vi "update_raps.vi"(8 "error in (no error)":errorcluster, 10 "settings cluster":T1={"number of pixels"=0, "iterations per pixel"=0, "iterations per subpixel"=0, "maximum bit-depth"=0, "AOD center freq. (Hz)"=0.0, "AOD bandwidth freq. (Hz)"=0.0, "AOD amplitude"=0, "pixel dwell time"=0.0, "AOD equilibration time"=65535.0, "ra trajectory pixels (data/pixels transfered)"=1, "pattern type"=-1, "ellipsoid parameter cluster"={"a"=0.0, "b"=0.0, "c"=0.0, "d"=0.0, "e"=0.0, "k"=0, "width"=0.0}, "pixel values cluster"={"channel 0"=0, "channel 1"=0, "channel 2"=0, "channel 3"=0}, "offset (Hz)"=[], "RAPS array"=[], "DDS board initialization parameters"={"Bypass PLL"=FALSE, "PLL Range"=FALSE, "Update Clock"=FALSE, "Triangle "=FALSE, "SDO Active"=FALSE, "LSB First"=FALSE, "OSK Int"=FALSE, "Output Shaped Keying Enable"=FALSE, "Bypass Sinc"=FALSE, "Digital Part"=FALSE, "OutPut DAC"=FALSE, "Control DAC"=FALSE, "Comparator"=FALSE, "Modus"=0, "Multiplier Value"=0}, "gates"=[]} {"ellipsoid parameter cluster"."a" format="%.16g"; "ellipsoid parameter cluster"."b" format="%.16g"; "ellipsoid parameter cluster"."c" format="%.16g"; "ellipsoid parameter cluster"."d" format="%.16g"; "DDS board initialization parameters"."Modus" scale=0.0..4.0}, 11 "FPGA VI Reference In":refnum<k20>) -> (0 "error out":errorcluster)   [LabVIEW 2010]
uses:
  <vilib>/rvi/interface/nirviReadWriteControl/nirviReadWriteControl.xnode
  <vilib>/rvi/interface/nirviMethod/nirviMethod.xnode
  common_typedefs/channels_cluster.ctl
  fpgaVIsAndControls/DDS_board_init_cluster.ctl
  FPGAWrapperMH120124RAPS_PXI7813R/settings_cluster_raps.ctl
  fpgaVIsAndControls/ellipsoid_parameters_cluster.ctl
  common_typedefs/gate_parameters_cluster.ctl
  fpgaVIsAndControls/gate_cluster.ctl
panel:
  # "FSK"
  # "Ramped"
  # "FSK"
  # "Chirp Modus"
  # "Unramped"
  # "BPSK"
  # "Single Tone"
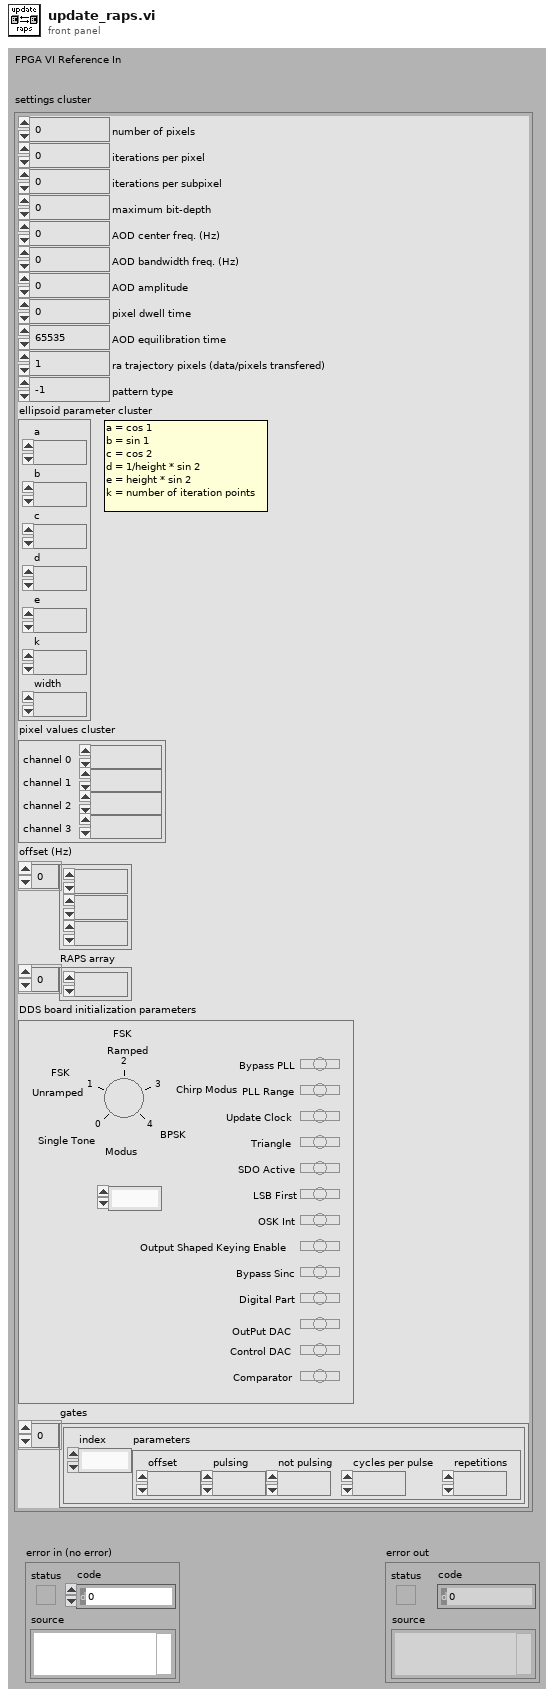
[diagram p1: front panel]
types:
  T1 = typedef "settings_cluster_raps.ctl" = cluster{"number of pixels":i32, "iterations per pixel":i32, "iterations per subpixel":i32, "maximum bit-depth":i8, "AOD center freq. (Hz)":dbl, "AOD bandwidth freq. (Hz)":dbl, "AOD amplitude":u16, "pixel dwell time":dbl, "AOD equilibration time":dbl, "ra trajectory pixels (data/pixels transfered)":u32, "pattern type":i8, "ellipsoid parameter cluster":T2, "pixel values cluster":T3, "offset (Hz)":dbl[], "RAPS array":u64[], "DDS board initialization parameters":T4, "gates":T5[]}
  T2 = typedef "ellipsoid_parameters_cluster.ctl" = cluster{"a":fxp<+/-,16,1>, "b":fxp<+/-,16,1>, "c":fxp<+/-,16,1>, "d":fxp<+/-,16,1>, "e":fxp<+/-,24,16>, "k":u16, "width":fxp<+,16,16>}
  T3 = typedef "channels_cluster.ctl" = cluster{"channel 0":u32, "channel 1":u32, "channel 2":u32, "channel 3":u32}
  T4 = typedef "DDS_board_init_cluster.ctl" = cluster{"Bypass PLL":bool, "PLL Range":bool, "Update Clock":bool, "Triangle ":bool, "SDO Active":bool, "LSB First":bool, "OSK Int":bool, "Output Shaped Keying Enable":bool, "Bypass Sinc":bool, "Digital Part":bool, "OutPut DAC":bool, "Control DAC":bool, "Comparator":bool, "Modus":u8, "Multiplier Value":u8}
  T5 = typedef "gate_cluster.ctl" = cluster{"index":i32, "parameters":T6}
  T6 = typedef "gate_parameters_cluster.ctl" = cluster{"offset":i64, "pulsing":i64, "not pulsing":i64, "cycles per pulse":i64, "repetitions":i64}
  T7 = cluster{"AOD Bandwidth_x (Hz)":fxp<+,36,32>, "AOD Bandwidth_y (Hz)":fxp<+,36,32>, "AOD half bandwidth_x":fxp<+,36,32>, "AOD half bandwidth_y":fxp<+,36,32>, "AOD_Scale_Factor (1/Zoom)":fxp<+,36,2>, "sin Phi":fxp<+/-,36,2>, "cos Phi":fxp<+/-,36,2>, "Bandwidth for LUTs (256pts)":fxp<+,36,0>, "AOD_Amplitude in":u16, "AOD center frequ. (Hz)_x":fxp<+,36,32>, "AOD center frequ. (Hz)_y":fxp<+,36,32>, "x offset (Hz)":fxp<+/-,36,32>, "y offset (Hz)":fxp<+/-,36,32>, "DA multiplier constant":fxp<+,64,4>}
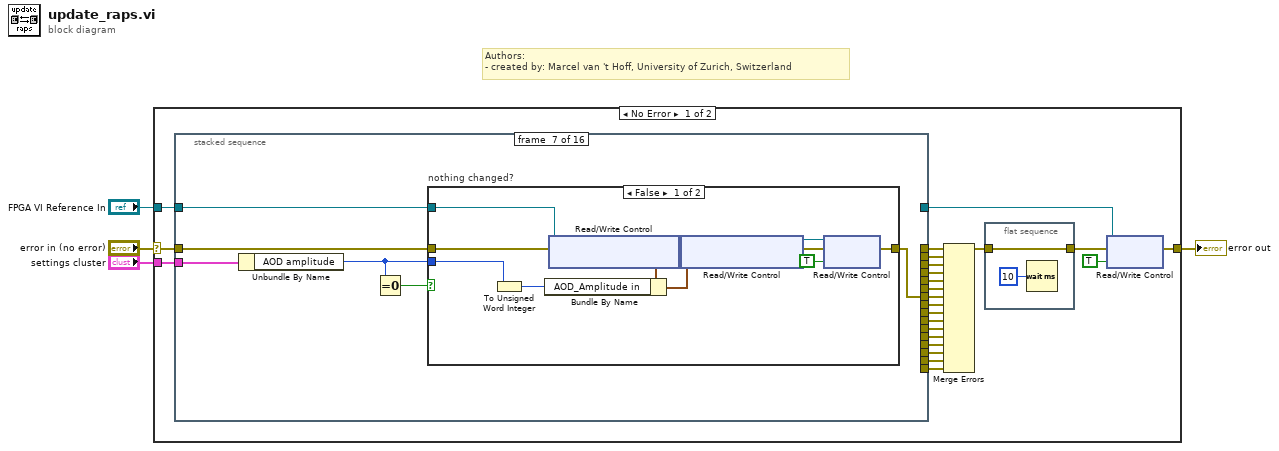
[diagram p0: block diagram]
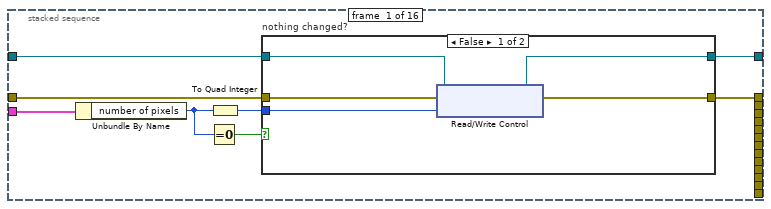
[diagram p2: hidden frame]
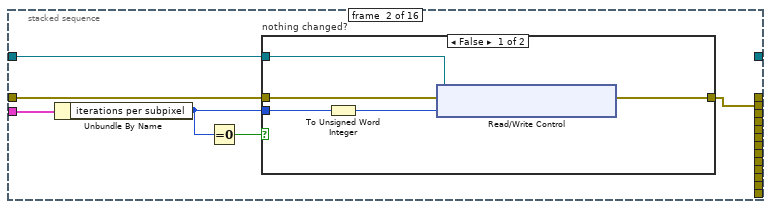
[diagram p4: hidden frame]
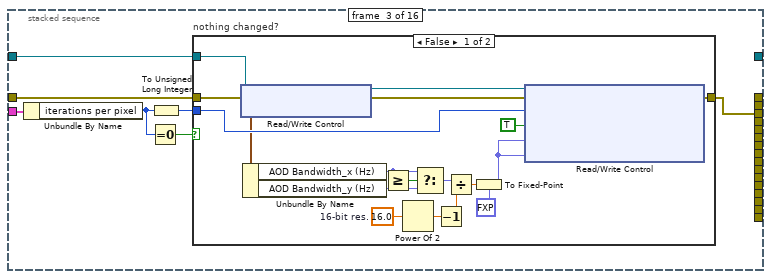
[diagram p6: hidden frame]
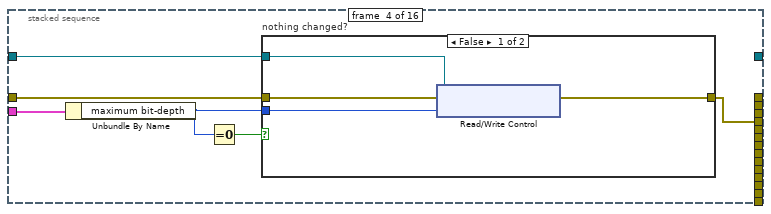
[diagram p8: hidden frame]
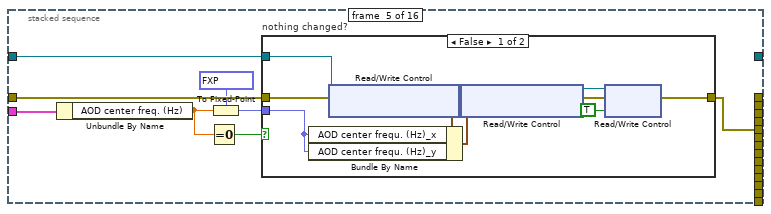
[diagram p10: hidden frame]
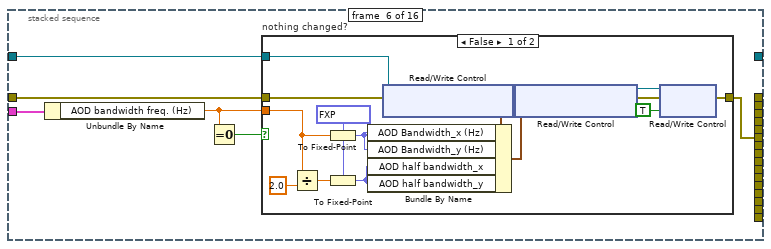
[diagram p12: hidden frame]
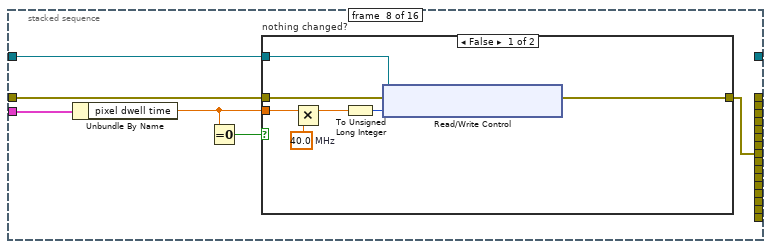
[diagram p15: hidden frame]
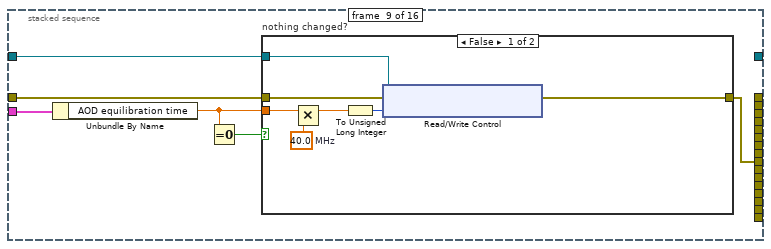
[diagram p17: hidden frame]
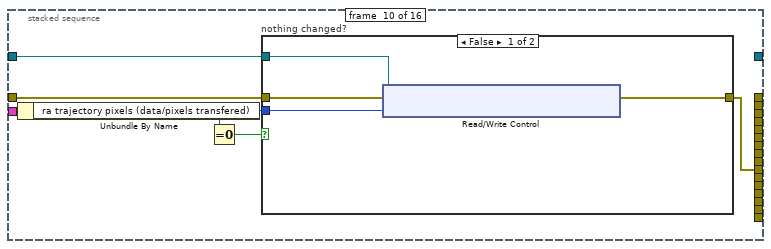
[diagram p19: hidden frame]
diagram:
  # "Authors: \n- created by: Marcel van 't Hoff, University of Zurich, Switzerland"
  n1 = case shown="No Error" "error in (no error)" {
    selector: "error in (no error)" -> [w15 w307]
    tunnel: "settings cluster" -> [w14 _]
    tunnel: "FPGA VI Reference In" -> [w16 _]
    tunnel: [w26 w307] -> w2
    frame No Error {
      n2 = stacked-sequence {
        tunnel: w14 -> [w36 w49 w62 w87 w100 w118 w141 w160 w174 w188 w200 w213 w225 w263 w274 w283]
        tunnel: [w30 _ _ _ _ _ _ _ _ _ _ _ _ _ _ _] -> w17
        tunnel: w15 -> [w32 w47 w58 w85 w98 w116 w139 w158 w172 w186 w198 w212 w224 w262 w273 w284]
        tunnel: w16 -> [w31 w46 w57 w84 w97 w115 w138 w157 w171 w185 w197 w211 w223 w261 w272 w282]
        tunnel: [_ _ w56 _ _ _ _ _ _ _ _ _ _ _ _ _] -> w18
        tunnel: [_ _ _ w82 _ _ _ _ _ _ _ _ _ _ _ _] -> w19
        tunnel: [_ _ _ _ w93 _ _ _ _ _ _ _ _ _ _ _] -> w20
        tunnel: [_ _ _ _ _ w113 _ _ _ _ _ _ _ _ _ _] -> w21
        tunnel: [_ _ _ _ _ _ w136 _ _ _ _ _ _ _ _ _] -> w22
        tunnel: [_ _ _ _ _ _ _ w155 _ _ _ _ _ _ _ _] -> w23
        tunnel: [_ _ _ _ _ _ _ _ _ _ w194 _ _ _ _ _] -> w24
        tunnel: [_ _ _ _ _ _ _ _ _ _ _ w206 _ _ _ _] -> w25
        tunnel: [w29 _ _ _ _ _ _ _ _ _ _ _ _ _ _ _] -> w12
        tunnel: [_ _ _ _ _ _ _ _ w169 _ _ _ _ _ _ _] -> w11
        tunnel: [_ _ _ _ _ _ _ _ _ w183 _ _ _ _ _ _] -> w10
        tunnel: [_ _ _ _ _ _ _ _ _ _ _ _ w219 _ _ _] -> w9
        tunnel: [_ _ _ _ _ _ _ _ _ _ _ _ _ w243 _ _] -> w8
        tunnel: [_ _ _ _ _ _ _ _ _ _ _ _ _ _ w270 _] -> w7
        tunnel: [_ w45 _ _ _ _ _ _ _ _ _ _ _ _ _ _] -> w6
        tunnel: [_ _ _ _ _ _ _ _ _ _ _ _ _ _ _ w281] -> w5
        frame #0 {
          n3 = Unbundle By Name(w36) -> ("number of pixels"=w35:i32)
          n4 = Equal To 0?(x=w35) -> (x = 0?=w34:bool)
          n5 = To Quad Integer(1:w35) -> (0:w33:i64)
          n6 = case "nothing changed?" shown="False" w34 {
            tunnel: w33 -> [w39 _]
            tunnel: [w41 w43] -> w30
            tunnel: w32 -> [w40 w43]
            tunnel: w31 -> [w38 w42]
            tunnel: [w37 w42] -> w29
            frame False {
              n7 = xnode "Read/Write Control"("FPGA VI Reference In"=w38, "error in"=w40, "number of pixels"=w39) -> ("FPGA VI Reference Out"=w37:refnum<k20>, "error out"=w41:errorcluster)
            }
            frame True {
              # "nothing changed"
            }
          }
        }
        frame #1 {
          n8 = Unbundle By Name(w49) -> ("iterations per subpixel"=w44:i32)
          n9 = Equal To 0?(x=w44) -> (x = 0?=w48:bool)
          n10 = case "nothing changed?" shown="False" w48 {
            tunnel: w44 -> [w51 _]
            tunnel: [w54 w55] -> w45
            tunnel: w47 -> [w53 w55]
            tunnel: w46 -> [w52 _]
            frame False {
              n11 = To Unsigned Word Integer(number=w51) -> (unsigned 16bit integer=w50:u16)
              n12 = xnode "Read/Write Control"("FPGA VI Reference In"=w52, "error in"=w53, "sub-pattern iterations per pixel"=w50) -> ("error out"=w54:errorcluster)  [unwired: 1 out]
            }
            frame True {
              # "nothing changed"
            }
          }
        }
        frame #2 {
          n13 = Unbundle By Name(w62) -> ("iterations per pixel"=w61:i32)
          n14 = Equal To 0?(x=w61) -> (x = 0?=w60:bool)
          n15 = To Unsigned Long Integer(number=w61) -> (unsigned 32bit integer=w59:u32)
          n16 = case "nothing changed?" shown="False" w60 {
            tunnel: w59 -> [w79 _]
            tunnel: [w80 w81] -> w56
            tunnel: w58 -> [w76 w81]
            tunnel: w57 -> [w78 _]
            frame False {
              w69 = 16.0  # 16-bit res.
              n17 = xnode "Read/Write Control"("FPGA VI Reference In"=w78, "error in"=w76) -> ("FPGA VI Reference Out"=w77:refnum<k20>, "error out"=w75:errorcluster, "FPGA parameters out"=w74:T7)
              n18 = Unbundle By Name(w74) -> ("AOD Bandwidth_x (Hz)"=w72:fxp<+,36,32>, "AOD Bandwidth_y (Hz)"=w71:fxp<+,36,32>)
              n19 = Greater Or Equal?(x=w72, y=w71) -> (x >= y?=w73:bool)
              n20 = Power Of 2(x=w69) -> (2^x=w68:dbl)
              n21 = Select(t=w72, s=w73, f=w71) -> (s? t:f=w70:fxp<+,36,32>)
              n22 = Decrement(x=w68) -> (x-1=w67:dbl)
              n23 = Divide(x=w70, y=w67) -> (x/y=w66:dbl)
              n24 = To Fixed-Point(fixed-point type=fxp<+,36,32> 0.0 ("AOD Bandwidth_x (Hz)"), number=w66) -> (fixed-point=w63:fxp<+,36,32>)
              n25 = xnode "Read/Write Control"("FPGA VI Reference In"=w77, "error in"=w75, "intergration iterations per pixel"=w79, "reset in"=TRUE, "x-point bandwidth"=w63, "y-point bandwidth"=w63) -> ("error out"=w80:errorcluster)  [unwired: 1 out]
            }
            frame True {
              # "nothing changed"
            }
          }
        }
        frame #3 {
          n26 = Unbundle By Name(w87) -> ("maximum bit-depth"=w83:i8)
          n27 = Equal To 0?(x=w83) -> (x = 0?=w86:bool)
          n28 = case "nothing changed?" shown="False" w86 {
            tunnel: w83 -> [w89 _]
            tunnel: [w91 w92] -> w82
            tunnel: w85 -> [w90 w92]
            tunnel: w84 -> [w88 _]
            frame False {
              n29 = xnode "Read/Write Control"("FPGA VI Reference In"=w88, "error in"=w90, "maximum bit depth"=w89) -> ("error out"=w91:errorcluster)  [unwired: 1 out]
            }
            frame True {
              # "nothing changed"
            }
          }
        }
        frame #4 {
          n30 = Unbundle By Name(w100) -> ("AOD center freq. (Hz)"=w95:dbl)
          n31 = Equal To 0?(x=w95) -> (x = 0?=w99:bool)
          n32 = To Fixed-Point(fixed-point type=fxp<+,36,32> 94000000.0 ("AOD center frequ. (MHz)"), number=w95) -> (fixed-point=w94:fxp<+,36,32>)
          n33 = case "nothing changed?" shown="False" w99 {
            tunnel: w94 -> [w105 _]
            tunnel: [w101 w112] -> w93
            tunnel: w98 -> [w109 w112]
            tunnel: w97 -> [w111 _]
            frame False {
              n34 = xnode "Read/Write Control"("FPGA VI Reference In"=w111, "error in"=w109) -> ("FPGA VI Reference Out"=w110:refnum<k20>, "error out"=w108:errorcluster, "FPGA parameters out"=w107:T7)
              n35 = Bundle By Name(cluster=w107, "AOD center frequ. (Hz)_x"=w105, "AOD center frequ. (Hz)_y"=w105) -> (w106:T7)
              n36 = xnode "Read/Write Control"("FPGA VI Reference In"=w110, "error in"=w108, "FPGA parameters in"=w106) -> ("FPGA VI Reference Out"=w103:refnum<k20>, "error out"=w102:errorcluster)
              n37 = xnode "Read/Write Control"("FPGA VI Reference In"=w103, "error in"=w102, "reset in"=TRUE) -> ("error out"=w101:errorcluster)  [unwired: 1 out]
            }
            frame True {
              # "nothing changed"
            }
          }
        }
        frame #5 {
          n38 = Unbundle By Name(w118) -> ("AOD bandwidth freq. (Hz)"=w114:dbl)
          n39 = Equal To 0?(x=w114) -> (x = 0?=w117:bool)
          n40 = case "nothing changed?" shown="False" w117 {
            tunnel: [w119 w135] -> w113
            tunnel: w116 -> [w132 w135]
            tunnel: w115 -> [w134 _]
            tunnel: w114 -> [w127 _]
            frame False {
              w124 = fxp<+,36,32> 35000000.0 ("AOD center frequ. (MHz)")
              n41 = Divide(x=w127, y=2.0) -> (x/y=w123:dbl)
              n42 = To Fixed-Point(fixed-point type=w124, number=w127) -> (fixed-point=w126:fxp<+,36,32>)
              n43 = To Fixed-Point(fixed-point type=w124, number=w123) -> (fixed-point=w125:fxp<+,36,32>)
              n44 = xnode "Read/Write Control"("FPGA VI Reference In"=w134, "error in"=w132) -> ("FPGA VI Reference Out"=w133:refnum<k20>, "error out"=w131:errorcluster, "FPGA parameters out"=w130:T7)
              n45 = Bundle By Name(cluster=w130, "AOD Bandwidth_x (Hz)"=w126, "AOD Bandwidth_y (Hz)"=w126, "AOD half bandwidth_x"=w125, "AOD half bandwidth_y"=w125) -> (w129:T7)
              n46 = xnode "Read/Write Control"("FPGA VI Reference In"=w133, "error in"=w131, "FPGA parameters in"=w129) -> ("FPGA VI Reference Out"=w121:refnum<k20>, "error out"=w120:errorcluster)
              n47 = xnode "Read/Write Control"("FPGA VI Reference In"=w121, "error in"=w120, "reset in"=TRUE) -> ("error out"=w119:errorcluster)  [unwired: 1 out]
            }
            frame True {
              # "nothing changed"
            }
          }
        }
        frame #6 {
          n48 = Unbundle By Name(w141) -> ("AOD amplitude"=w137:u16)
          n49 = Equal To 0?(x=w137) -> (x = 0?=w140:bool)
          n50 = case "nothing changed?" shown="False" w140 {
            tunnel: [w142 w154] -> w136
            tunnel: w139 -> [w151 w154]
            tunnel: w138 -> [w153 _]
            tunnel: w137 -> [w147 _]
            frame False {
              n51 = To Unsigned Word Integer(number=w147) -> (unsigned 16bit integer=w146:u16)
              n52 = xnode "Read/Write Control"("FPGA VI Reference In"=w153, "error in"=w151) -> ("FPGA VI Reference Out"=w152:refnum<k20>, "error out"=w150:errorcluster, "FPGA parameters out"=w149:T7)
              n53 = Bundle By Name(cluster=w149, "AOD_Amplitude in"=w146) -> (w148:T7)
              n54 = xnode "Read/Write Control"("FPGA VI Reference In"=w152, "error in"=w150, "FPGA parameters in"=w148) -> ("FPGA VI Reference Out"=w143:refnum<k20>, "error out"=w144:errorcluster)
              n55 = xnode "Read/Write Control"("FPGA VI Reference In"=w143, "error in"=w144, "reset in"=TRUE) -> ("error out"=w142:errorcluster)  [unwired: 1 out]
            }
            frame True {
              # "nothing changed"
            }
          }
        }
        frame #7 {
          n56 = Unbundle By Name(w160) -> ("pixel dwell time"=w156:dbl)
          n57 = Equal To 0?(x=w156) -> (x = 0?=w159:bool)
          n58 = case "nothing changed?" shown="False" w159 {
            tunnel: [w162 w168] -> w155
            tunnel: w158 -> [w166 w168]
            tunnel: w157 -> [w167 _]
            tunnel: w156 -> [w165 _]
            frame False {
              w164 = 40.0  # MHz
              n59 = Multiply(x=w165, y=w164) -> (x*y=w163:dbl)
              n60 = To Unsigned Long Integer(number=w163) -> (unsigned 32bit integer=w161:u32)
              n61 = xnode "Read/Write Control"("FPGA VI Reference In"=w167, "error in"=w166, "intergration iterations per pixel"=w161) -> ("error out"=w162:errorcluster)  [unwired: 1 out]
            }
            frame True {
              # "nothing changed"
            }
          }
        }
        frame #8 {
          n62 = Unbundle By Name(w174) -> ("AOD equilibration time"=w170:dbl)
          n63 = Equal To 0?(x=w170) -> (x = 0?=w173:bool)
          n64 = case "nothing changed?" shown="False" w173 {
            tunnel: [w176 w182] -> w169
            tunnel: w172 -> [w180 w182]
            tunnel: w171 -> [w181 _]
            tunnel: w170 -> [w179 _]
            frame False {
              w178 = 40.0  # MHz
              n65 = Multiply(x=w179, y=w178) -> (x*y=w177:dbl)
              n66 = To Unsigned Long Integer(number=w177) -> (unsigned 32bit integer=w175:u32)
              n67 = xnode "Read/Write Control"("FPGA VI Reference In"=w181, "error in"=w180, "waiting iterations  per pixel"=w175) -> ("error out"=w176:errorcluster)  [unwired: 1 out]
            }
            frame True {
              # "nothing changed"
            }
          }
        }
        frame #9 {
          n68 = Unbundle By Name(w188) -> ("ra trajectory pixels (data/pixels transfered)"=w184:u32)
          n69 = Equal To 0?(x=w184) -> (x = 0?=w187:bool)
          n70 = case "nothing changed?" shown="False" w187 {
            tunnel: [w190 w193] -> w183
            tunnel: w186 -> [w191 w193]
            tunnel: w185 -> [w192 _]
            tunnel: w184 -> [w189 _]
            frame False {
              n71 = xnode "Read/Write Control"("FPGA VI Reference In"=w192, "error in"=w191, "ra trajectory pixels (data/pixels transfered)"=w189) -> ("error out"=w190:errorcluster)  [unwired: 1 out]
            }
            frame True {
              # "nothing changed"
            }
          }
        }
        frame #10 {
          n72 = Unbundle By Name(w200) -> ("ellipsoid parameter cluster"=w196:T2, "ellipsoid parameter cluster.k"=w195:u16)
          n73 = Equal To 0?(x=w195) -> (x = 0?=w199:bool)
          n74 = case "nothing changed?" shown="False" w199 {
            tunnel: [w202 w205] -> w194
            tunnel: w198 -> [w203 w205]
            tunnel: w197 -> [w204 _]
            tunnel: w196 -> [w201 _]
            frame False {
              n75 = xnode "Read/Write Control"("FPGA VI Reference In"=w204, "error in"=w203, "ellipsoid parameter cluster"=w201) -> ("error out"=w202:errorcluster)  [unwired: 1 out]
            }
            frame True {
              # "nothing changed"
            }
          }
        }
        frame #11 {
          n76 = Unbundle By Name(w213) -> ("pixel values cluster"=w210:T3)
          n77 = Cluster To Array(cluster=w210) -> (array=w208:u32[])
          n78 = Add Array Elements(numeric array=w208) -> (sum=w207:u32)
          n79 = Equal To 0?(x=w207) -> (x = 0?=w209:bool)
          n80 = case "nothing changed?" shown="False" w209 {
            tunnel: [w215 w218] -> w206
            tunnel: w212 -> [w216 w218]
            tunnel: w211 -> [w217 _]
            tunnel: w210 -> [w214 _]
            frame False {
              n81 = xnode "Read/Write Control"("FPGA VI Reference In"=w217, "error in"=w216, "channel offsets"=w214) -> ("error out"=w215:errorcluster)  [unwired: 1 out]
            }
            frame True {
              # "nothing changed"
            }
          }
        }
        frame #12 {
          n82 = Unbundle By Name(w225) -> ("offset (Hz)"=w220:dbl[])
          n83 = Add Array Elements(numeric array=w220) -> (sum=w221:dbl)
          n84 = Equal To 0?(x=w221) -> (x = 0?=w222:bool)
          n85 = case "nothing changed?" shown="False" w222 {
            tunnel: [w226 w242] -> w219
            tunnel: w224 -> [w240 w242]
            tunnel: w223 -> [w241 _]
            tunnel: w220 -> [w238 _]
            frame False {
              w239 = fxp<+/-,36,32> 0.0 ("x offset (Hz)")
              n86 = Index Array(array=w238) -> (element #1=w237:dbl, element #2=w236:dbl)  [unwired: 2 in]
              n87 = To Fixed-Point(fixed-point type=w239, number=w237) -> (fixed-point=w231:fxp<+/-,36,32>)
              n88 = To Fixed-Point(fixed-point type=w239, number=w236) -> (fixed-point=w230:fxp<+/-,36,32>)
              n89 = xnode "Read/Write Control"("FPGA VI Reference In"=w241, "error in"=w240) -> ("FPGA VI Reference Out"=w235:refnum<k20>, "error out"=w234:errorcluster, "FPGA parameters out"=w233:T7)
              n90 = Bundle By Name(cluster=w233, "x offset (Hz)"=w231, "y offset (Hz)"=w230) -> (w232:T7)
              n91 = xnode "Read/Write Control"("FPGA VI Reference In"=w235, "error in"=w234, "FPGA parameters in"=w232) -> ("FPGA VI Reference Out"=w227:refnum<k20>, "error out"=w228:errorcluster)
              n92 = xnode "Read/Write Control"("FPGA VI Reference In"=w227, "error in"=w228, "reset in"=TRUE) -> ("error out"=w226:errorcluster)  [unwired: 1 out]
            }
            frame True {
              # "nothing changed"
            }
          }
        }
        frame #13 {
          n93 = Unbundle By Name(w263) -> ("DDS board initialization parameters"=w260:T4)
          n94 = Unbundle(w260) -> ("Bypass PLL"=w259:bool, "PLL Range"=w258:bool, "Update Clock"=w257:bool, "Triangle"=w256:bool, "SDO Active"=w255:bool, "LSB First"=w254:bool, "OSK Int"=w253:bool, "Output Shaped Keying Enable"=w252:bool, "Bypass Sinc"=w251:bool, "Digital Part"=w250:bool, "OutPut DAC"=w249:bool, "Control DAC"=w248:bool, "Comparator"=w247:bool)  [unwired: 2 out]
          n95 = Build Array(w259, w258, w257, w256, w255, w254, w253, w252, w251, w250, w249, w248, w247) -> (w246:bool[])
          n96 = Boolean Array To Number(Boolean array=w246) -> (number=w244:u32)
          n97 = Equal To 0?(x=w244) -> (x = 0?=w245:bool)
          n98 = case "nothing changed?" shown="False" w245 {
            tunnel: [w265 w268] -> w243
            tunnel: w262 -> [w266 w268]
            tunnel: w261 -> [w267 _]
            tunnel: w260 -> [w264 _]
            frame False {
              n99 = xnode "Read/Write Control"("FPGA VI Reference In"=w267, "error in"=w266, "DDS board initialization parameters"=w264) -> ("error out"=w265:errorcluster)  [unwired: 1 out]
            }
            frame True {
              # "nothing changed"
            }
          }
        }
        frame #14 {
          n100 = Unbundle By Name(w274) -> ("RAPS array"=w269:u64[])
          n101 = Empty Array?(array=w269) -> (empty?=w271:bool)
          n102 = case "nothing changed?" shown="False" w271 {
            tunnel: [w276 w280] -> w270
            tunnel: w273 -> [w277 w280]
            tunnel: w272 -> [w279 _]
            tunnel: w269 -> [w278 _]
            frame False {
              n103 = xnode "Invoke Method"("FPGA VI Reference In"=w279, "error in"=w277, "Data"=w278, "Timeout (ms)"=5000) -> ("error out"=w276:errorcluster)  [unwired: 2 out]
            }
            frame True {
              # "nothing changed"
            }
          }
        }
        frame #15 {
          n104 = Unbundle By Name(w283) -> ("gates"=w285:T5[])
          n105 = for "Loop over specified gates..." {
            tunnel: w285 -> [w291] mode=indexing
            tunnel: w282 -> [w290]
            shift-right: [w288] -> w281
            shift-left: w284 -> [w289]
            stop <- w288 stop-if-true
            n106 = Unbundle By Name(w291) -> ("index"=w286:i32, "parameters"=w287:T6)
            n107 = case "Which gate?" shown="Default" w286 {
              tunnel: w290 -> [_ w296 w297 w304]
              tunnel: w289 -> [w292 w295 w300 w303]
              tunnel: [w292 w294 w299 w301] -> w288
              tunnel: w287 -> [_ w293 w298 w302]
              frame Default {
              }
              frame 1 {
                n108 = xnode "Read/Write Control"("FPGA VI Reference In"=w296, "error in"=w295, "gate 1"=w293) -> ("error out"=w294:errorcluster)  [unwired: 1 out]
              }
              frame 2 {
                n109 = xnode "Read/Write Control"("FPGA VI Reference In"=w297, "error in"=w300, "gate 2"=w298) -> ("error out"=w299:errorcluster)  [unwired: 1 out]
              }
              frame 3 {
                n110 = xnode "Read/Write Control"("FPGA VI Reference In"=w304, "error in"=w303, "gate 3"=w302) -> ("error out"=w301:errorcluster)  [unwired: 1 out]
              }
            }
          }
        }
      }
      n111 = Merge Errors(w17, w6, w18, w19, w20, w21, w22, w23, w11, w10, w24, w25, w9, w8, w7, w5) -> (w13:errorcluster)
      n112 = flat-sequence {
        tunnel: [w305] -> w28
        tunnel: w13 -> [w305]
        frame #0 {
          n113 = Wait (ms)(milliseconds to wait=u32 10) -> ()  [unwired: 1 out]
        }
      }
      n114 = xnode "Read/Write Control"("FPGA VI Reference In"=w12, "error in"=w28, "reset in"=TRUE) -> ("error out"=w26:errorcluster)  [unwired: 1 out]
    }
    frame Error {
    }
  }
  "error out" <- w2
